vi "knightRider.vi"(10 "String":string="1") -> ()   [LabVIEW 2013]
uses:
  TestGlobal.vi
panel:
  out "String 2":string
  out "Numerisch":u32
  out "Array":bool[](array[boolean])=[FALSE, FALSE, FALSE, FALSE, TRUE, FALSE, FALSE, FALSE]
  in  "stop":bool
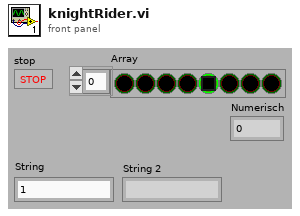
[diagram p1: front panel]
types:
  T1 = enum32{"invalid app kind", "Development System", "Run Time System", "Student Edition", "Embedded LabVIEW", "Evaluation", "Custom"}
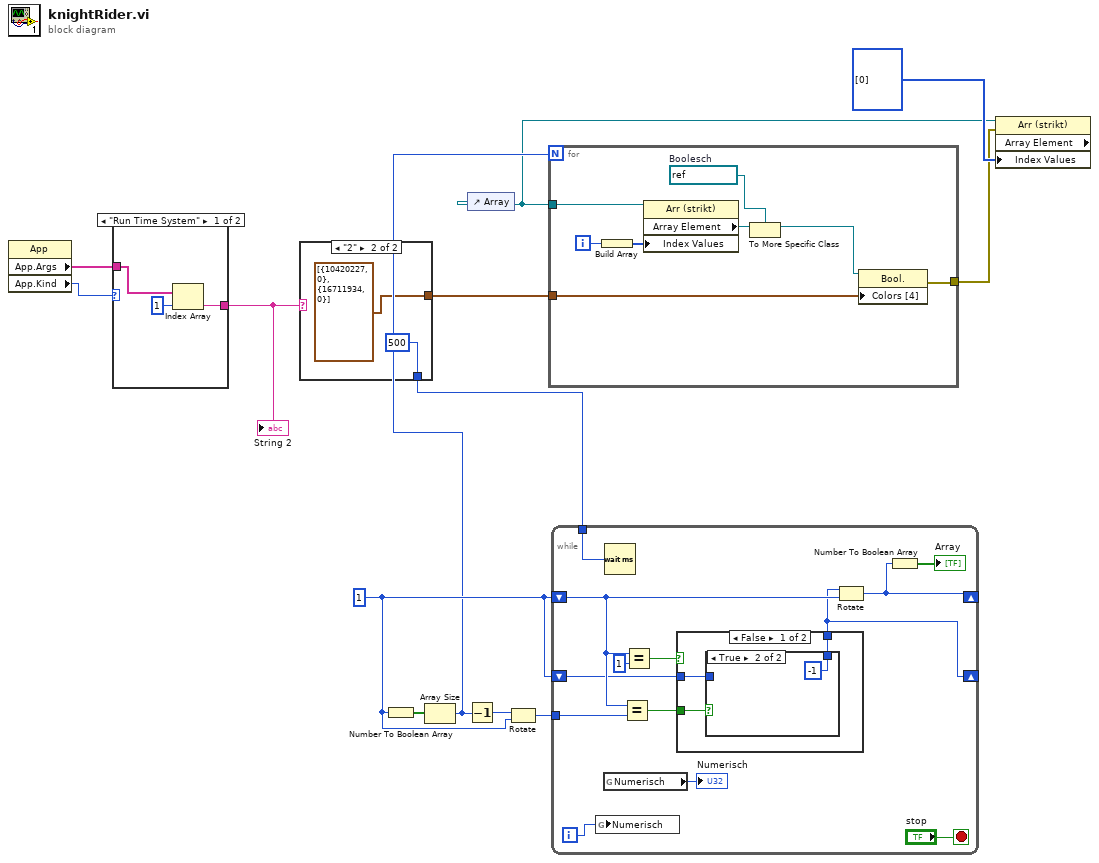
[diagram p0: block diagram]
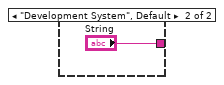
[diagram p2: hidden frame]
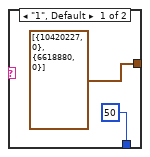
[diagram p3: hidden frame]
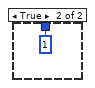
[diagram p5: hidden frame]
diagram:
  w10 = u8 1 ("y")
  n1 = property class="App"() -> ("App.Args"=w1:string[], "App.Kind"=w2:T1)  [unwired: 2 in, 2 out]
  n2 = case shown="\"Run Time System\"" w2 {
    tunnel: [w14 "String"] -> w8
    tunnel: w1 -> [w16 _]
    frame "Run Time System" {
      n3 = Index Array(array=w16, index=1 ("Index")) -> (element=w14:string)
    }
    frame "Development System", Default {
    }
  }
  "String 2" <- w8
  n4 = case shown="\"2\"" w8 {
    tunnel: [cluster{u32, u32}[] [{10420227, 0}, {6618880, 0}] ("Farben [4]") cluster{u32, u32}[] [{10420227, 0}, {16711934, 0}] ("Farben [4]")] -> w7
    tunnel: [u32 50 ("milliseconds to wait") 500] -> w6
    frame "1", Default {
    }
    frame "2" {
    }
  }
  n5 = Number To Boolean Array(number=w10) -> (Boolean array=w13:bool[])
  n6 = Array Size(array=w13) -> (size(s)=w9:i32)
  n7 = Decrement(x=w9) -> (x-1=w11:i32)
  n8 = control-ref of="Array"() -> (w4:refnum<vi>)
  n9 = Rotate(1:w10, 2:w11) -> (0:w12:u8)
  n10 = for {
    N: w9 -> [_]
    tunnel: w4 -> [w29]
    tunnel: w7 -> [w23]
    tunnel: [w22] -> w3
    i -> [w28]
    w24 = refnum<vi> refnum  # Boolesch
    n11 = Build Array(w28) -> (w27:i32[])
    n12 = property class="Arr (strikt)"(reference=w29, "Index Values"=w27) -> ("Array Element"=w26:refnum<vi>)  [unwired: 1 in, 2 out]
    n13 = To More Specific Class(target class=w24, reference=w26) -> (specific class reference=w25:refnum<vi>)  [unwired: 1 in, 1 out]
    n14 = property class="Bool."(reference=w25, "Colors [4]"=w23) -> (error out=w22:errorcluster)  [unwired: 1 in, 1 out]
  }
  n15 = while {
    shift-right: [w40] -> _
    shift-left: w10 -> [w37]
    tunnel: w12 -> [w35]
    shift-right: [w33] -> _
    shift-left: w10 -> [w34]
    tunnel: w6 -> [w32]
    i -> [w31]
    stop <- "stop" stop-if-true
    n16 = global write "TestGlobal.vi" "Numerisch"(w31) -> ()
    n17 = global read "TestGlobal.vi" "Numerisch"() -> (→"Numerisch":u32)
    n18 = Wait (ms)(milliseconds to wait=w32) -> ()  [unwired: 1 out]
    n19 = Equal?(x=w37, y=w35) -> (x = y?=w39:bool)
    n20 = Equal?(x=w37, y=u8 1) -> (x = y?=w38:bool)
    n21 = case shown="False" w38 {
      tunnel: w39 -> [w45 _]
      tunnel: [w44 i8 1 ("t")] -> w33
      tunnel: w34 -> [w43 _]
      frame False {
        n22 = case shown="True" w45 {
          tunnel: [w46 i8 -1 ("t")] -> w44
          tunnel: w43 -> [w46 _]
          frame False {
          }
          frame True {
          }
        }
      }
      frame True {
      }
    }
    n23 = Rotate(1:w37, 2:w33) -> (0:w40:u8)
    n24 = Number To Boolean Array(number=w40) -> (Boolean array=→"Array":bool[])
  }
  n25 = property class="Arr (strikt)" props=["Array Element", "Index Values"](reference=w4, error in=w3, "Index Values"=u32[] [0] ("Indexwerte")) -> ()  [unwired: 3 out]
